vi "decrementNofThreads.vi"(0 "HGF_ThreadPool":refnum<class "HGF_ThreadPool.lvclass">, 2 "threadRef":refnum<vi>, 5 "error in (no error)":errorcluster) -> (14 "dup HGF_ThreadPool":refnum<class "HGF_ThreadPool.lvclass">, 19 "error out":errorcluster)   [LabVIEW 2014, in "HGF_BaseClasses.lvlib" / "HGF_ThreadPool.lvclass"]
doc: "Decrement number of active threads and remove thread reference.\n\n<b>Attention:</b> This VI should be call from HGF_ThreadWorker.thread.vi only!"
uses:
  HGF_ThreadPool.lvclass
  HGF_Auxiliary/HGF_Auxiliary.lvlib
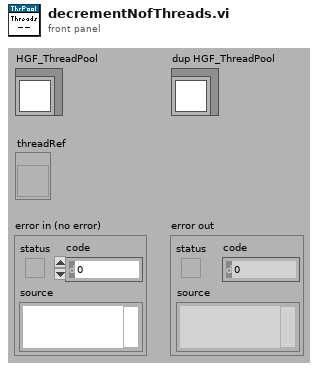
[diagram p1: front panel]
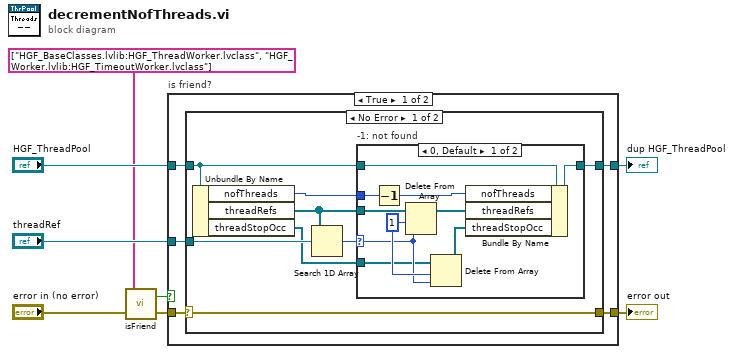
[diagram p0: block diagram]
diagram:
  n1 = call "isFriend.vi"("error in (no error)"="error in (no error)", "Friends"=string[] ["HGF_BaseClasses.lvlib:HGF_ThreadWorker.lvclass", "HGF_Worker.lvlib:HGF_TimeoutWorker.lvclass"]) -> ("error out"=w3:errorcluster, "isFriend?"=w2:bool)
  n2 = case "is friend?" shown="True" w2 {
    tunnel: w3 -> [w13 w35]
    tunnel: [w12 w35] -> w8
    tunnel: "HGF_ThreadPool" -> [w11 w36]
    tunnel: [w10 w36] -> w6
    tunnel: "threadRef" -> [w9 _]
    frame True {
      n3 = case shown="No Error" w13 {
        selector: w13 -> [w21 w33]
        tunnel: [w21 w33] -> w12
        tunnel: [w19 w34] -> w10
        tunnel: w11 -> [w20 w34]
        tunnel: w9 -> [w17 _]
        frame No Error {
          n4 = Unbundle By Name(w20) -> ("nofThreads"=w18:i32, "threadRefs"=w16:refnum<vi>[], "threadStopOcc"=w14:refnum<k4>[])
          n5 = Search 1D Array(1D array=w16, element=w17) -> (index of element=w15:i32)  [unwired: 1 out]
          n6 = case "-1: not found" shown="0, Default" w15 {
            selector: w15 -> [w24 _]
            tunnel: w20 -> [w31 w32]
            tunnel: [w30 w32] -> w19
            tunnel: w18 -> [w29 _]
            tunnel: w16 -> [w27 _]
            tunnel: w14 -> [w23 _]
            frame 0, Default {
              w25 = 1 ("length")
              n7 = Decrement(x=w29) -> (x-1=w28:i32)
              n8 = Delete From Array(array=w27, length=w25, index=w24) -> (array with subset deleted=w26:refnum<vi>[])  [unwired: 1 out]
              n9 = Delete From Array(array=w23, length=w25, index=w24) -> (array with subset deleted=w22:refnum<k4>[])  [unwired: 1 out]
              n10 = Bundle By Name(cluster=w31, "nofThreads"=w28, "threadRefs"=w26, "threadStopOcc"=w22) -> (w30:refnum<class "HGF_ThreadPool.lvclass">)
            }
            frame -1 {
            }
          }
        }
        frame Error {
        }
      }
    }
    frame False {
    }
  }
  "error out" <- w8
  "dup HGF_ThreadPool" <- w6
